vi "Polar Plat PG angle.vi"(4 "axis labels":string[](array[string])=["", "90", "180", "270"], 5 "desired font(Application)":T4(ring)=enum."Application Font", 6 "grid measurements":T1, 7 "[user-specified font]":T3, 11 "picture  in":picture) -> (3 "picture  out":picture)   [LabVIEW 2020]
panel:
  in  "label justification":T2(array[cluster])=[{"horizontal"=enum."right", "vertical"=enum."bottom"}, {"horizontal"=enum."left", "vertical"=enum."bottom"}, {"horizontal"=enum."left", "vertical"=enum."top"}, {"horizontal"=enum."right", "vertical"=enum."top"}]
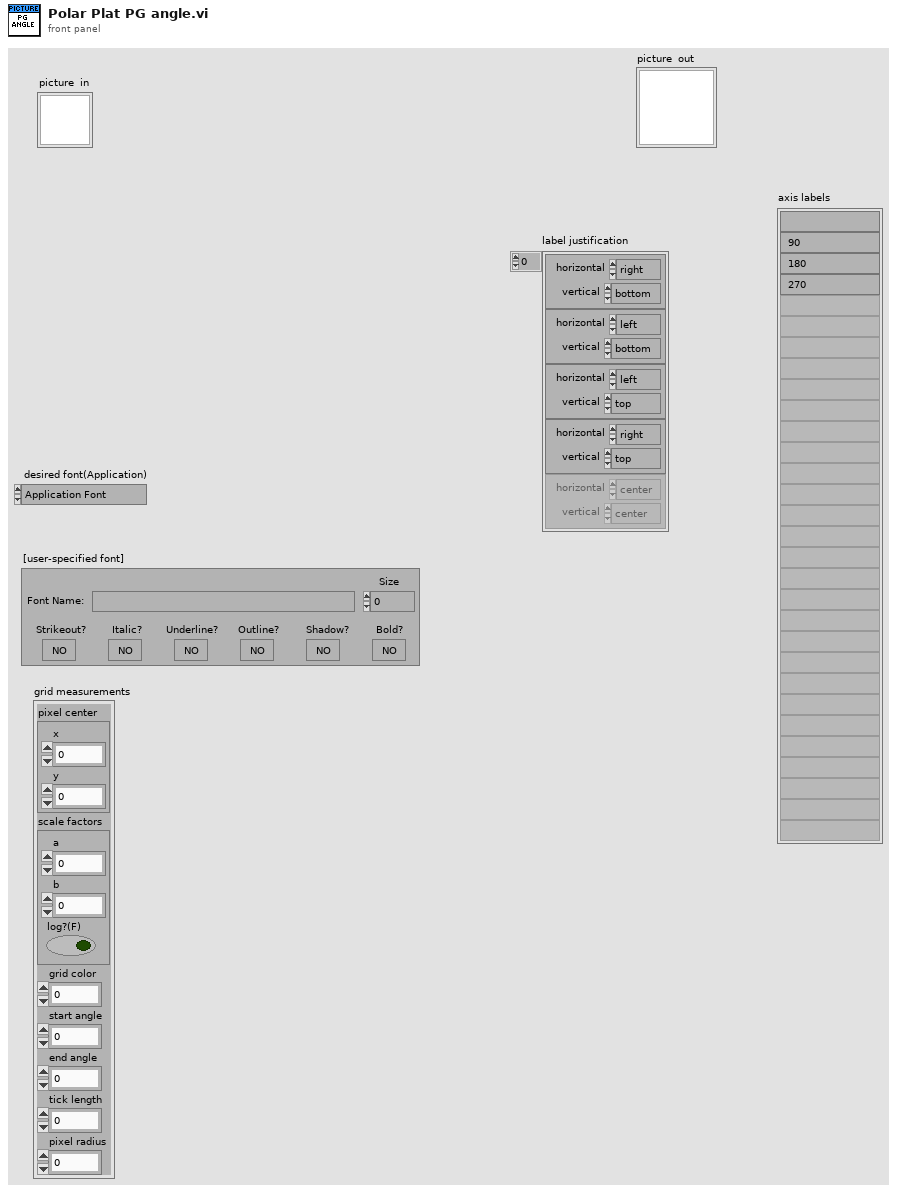
[diagram p1: front panel]
types:
  T1 = cluster{"pixel center":cluster{"x":i16, "y":i16}, "scale factors":cluster{"a":dbl, "b":dbl, "log?(F)":bool}, "grid color":u32, "start angle":dbl, "end angle":dbl, "tick length":i16, "pixel radius":i32}
  T2 = cluster{"horizontal":enum16{"left", "center", "right"}, "vertical":enum16{"top", "center", "bottom"}}[]
  T3 = cluster{"Font Name:":string, "Size":i16, "Strikeout?":bool, "Italic?":bool, "Underline?":bool, "Outline?":bool, "Shadow?":bool, "Bold?":bool}
  T4 = enum16{"User-specified Font", "Application Font", "System Font", "Dialog Font"}
  T5 = cluster{"horizontal":enum16{"left", "center", "right"}, "vertical":enum16{"top", "center", "bottom"}}
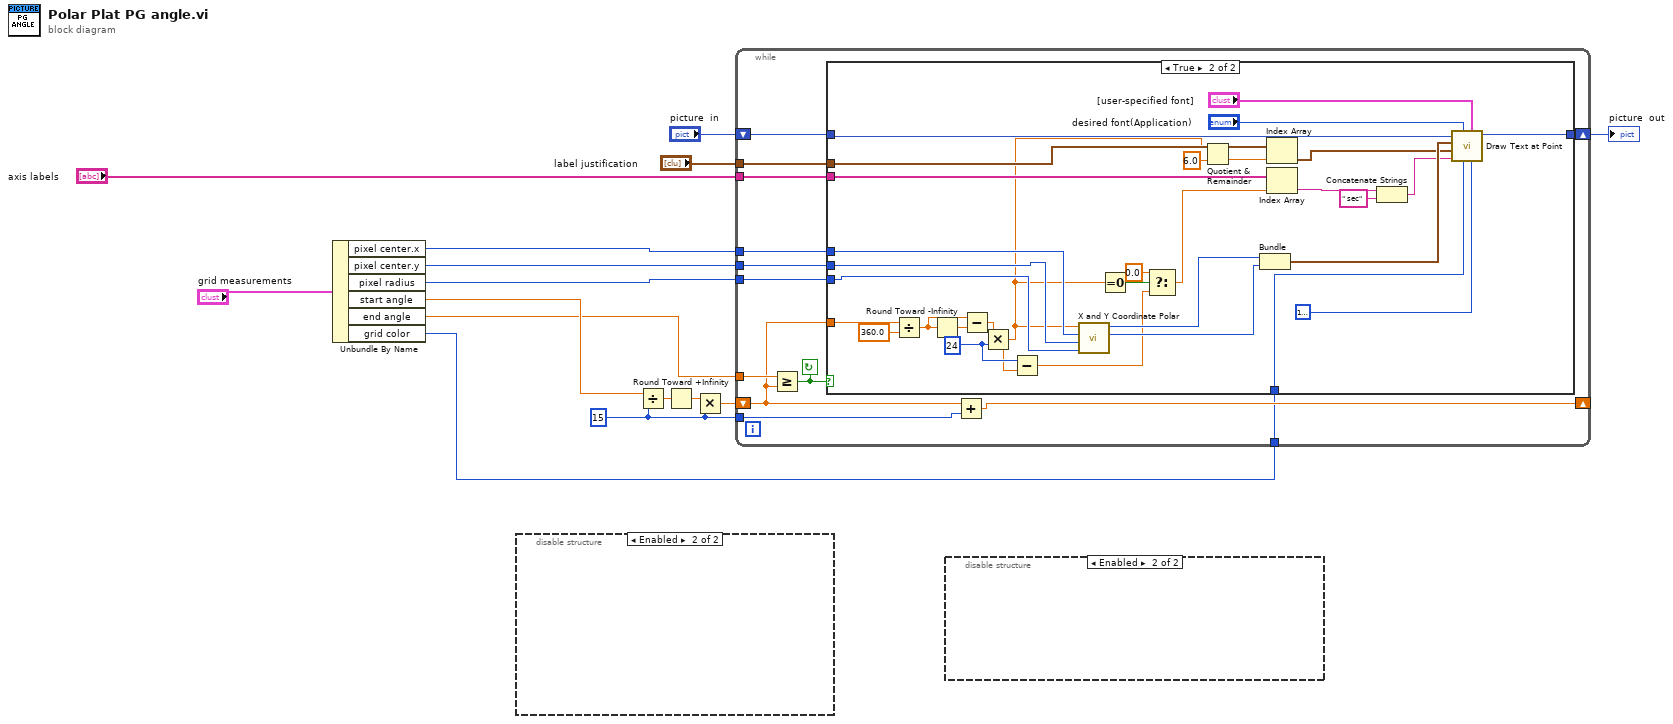
[diagram p0: block diagram]
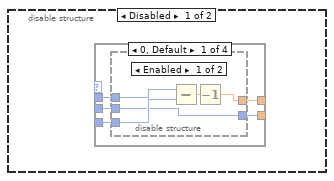
[diagram p2: hidden frame]
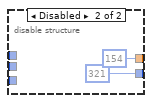
[diagram p3: hidden frame]
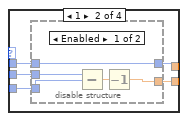
[diagram p4: hidden frame]
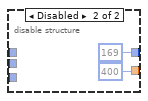
[diagram p5: hidden frame]
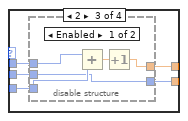
[diagram p6: hidden frame]
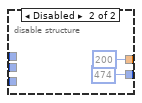
[diagram p7: hidden frame]
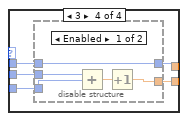
[diagram p8: hidden frame]
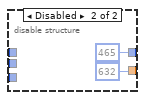
[diagram p9: hidden frame]
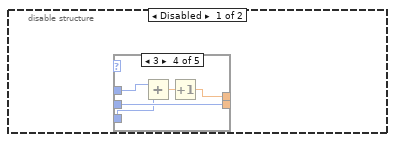
[diagram p10: hidden frame]
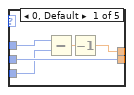
[diagram p11: hidden frame]
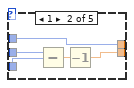
[diagram p12: hidden frame]
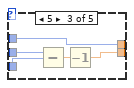
[diagram p13: hidden frame]
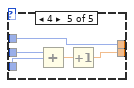
[diagram p14: hidden frame]
diagram:
  w9 = 15
  n1 = Unbundle By Name("grid measurements") -> ("pixel center.x"=w14:i16, "pixel center.y"=w13:i16, "pixel radius"=w12:i32, "start angle"=w11:dbl, "end angle"=w10:dbl, "grid color"=w15:u32)
  n2 = disable-structure shown="Enabled" {
    frame Disabled {
      n3 = case shown="0, Default" {
        selector: _ -> [_ _ _ _]
        tunnel: _ -> [w20 w29 w44 w53]
        tunnel: _ -> [w17 w32 w41 w56]
        tunnel: [w19 w28 w43 w52] -> _
        tunnel: [w16 w31 w40 w55] -> _
        tunnel: _ -> [w18 w30 w42 w54]
        frame 0, Default {
          n4 = disable-structure shown="Enabled" {
            disable-tunnel: w20 -> [w25 _]
            disable-tunnel: [w23 154] -> w19
            disable-tunnel: w18 -> [w22 _]
            disable-tunnel: w17 -> [w21 _]
            disable-tunnel: [w21 i16 321 ("y")] -> w16
            frame Enabled {
              n5 = Subtract(x=w25, y=w22) -> (x-y=w24:dbl)
              n6 = Decrement(x=w24) -> (x-1=w23:dbl)
            }
            frame Disabled {
            }
          }
        }
        frame 1 {
          n7 = disable-structure shown="Enabled" {
            disable-tunnel: w32 -> [w37 _]
            disable-tunnel: [w35 400] -> w31
            disable-tunnel: w30 -> [w34 _]
            disable-tunnel: w29 -> [w33 _]
            disable-tunnel: [w33 i16 169 ("x")] -> w28
            frame Enabled {
              n8 = Subtract(x=w37, y=w34) -> (x-y=w36:dbl)
              n9 = Decrement(x=w36) -> (x-1=w35:dbl)
            }
            frame Disabled {
            }
          }
        }
        frame 2 {
          n10 = disable-structure shown="Enabled" {
            disable-tunnel: w44 -> [w48 _]
            disable-tunnel: [w47 200] -> w43
            disable-tunnel: w42 -> [w46 _]
            disable-tunnel: w41 -> [w45 _]
            disable-tunnel: [w45 i16 474 ("y")] -> w40
            frame Enabled {
              n11 = Add(x=w48, y=w46) -> (x+y=w49:dbl)
              n12 = Increment(x=w49) -> (x+1=w47:dbl)
            }
            frame Disabled {
            }
          }
        }
        frame 3 {
          n13 = disable-structure shown="Enabled" {
            disable-tunnel: w56 -> [w61 _]
            disable-tunnel: [w59 632] -> w55
            disable-tunnel: w54 -> [w58 _]
            disable-tunnel: w53 -> [w57 _]
            disable-tunnel: [w57 i16 465 ("x")] -> w52
            frame Enabled {
              n14 = Add(x=w61, y=w58) -> (x+y=w60:dbl)
              n15 = Increment(x=w60) -> (x+1=w59:dbl)
            }
            frame Disabled {
            }
          }
        }
      }
    }
    frame Enabled {
    }
  }
  n16 = Divide(x=w11, y=w9) -> (x/y=w6:dbl)
  n17 = Round Toward +Infinity(x=w6) -> (ceil(x): smallest int >= x=w7:dbl)
  n18 = Multiply(x=w7, y=w9) -> (x*y=w8:dbl)
  n19 = while {
    tunnel: w14 -> [w67]
    tunnel: w13 -> [w68]
    tunnel: w12 -> [w69]
    shift-left: "picture  in" -> [w70]
    shift-right: [w71] -> w4
    tunnel: w10 -> [w75]
    tunnel: w9 -> [w76]
    shift-left: w8 -> [w72]
    shift-right: [w74] -> _
    tunnel: w15 -> [w66]
    tunnel: "axis labels" -> [w65]
    tunnel: "label justification" -> [w64]
    stop <- w73 continue-if-true
    n20 = Greater Or Equal?(x=w75, y=w72) -> (x >= y?=w73:bool)
    n21 = case shown="True" w73 {
      tunnel: w72 -> [_ w106]
      tunnel: [w77 w103] -> w71
      tunnel: w70 -> [w77 w102]
      tunnel: w69 -> [_ w91]
      tunnel: w68 -> [_ w92]
      tunnel: w67 -> [_ w93]
      tunnel: w66 -> [_ w99]
      tunnel: w65 -> [_ w87]
      tunnel: w64 -> [_ w86]
      frame False {
      }
      frame True {
        w88 = 24
        n22 = Divide(x=w106, y=360.0) -> (x/y=w98:dbl)
        n23 = Round Toward -Infinity(1:w98) -> (0:w108:dbl)
        n24 = Subtract(x=w98, y=w108) -> (x-y=w97:dbl)
        n25 = Multiply(x=w97, y=w88) -> (x*y=w82:dbl)
        n26 = Subtract(x=w88, y=w82) -> (x-y=w78:dbl)
        n27 = call "X and Y Coordinate Polar.vi"("Rc"=w91, "Yc"=w92, "Xc"=w93, "Selected Coordinate"=w82) -> ("Youtput"=w89:u32, "Xoutput"=w90:u32)  [unwired: 5 in, 1 out]
        n28 = Equal To 0?(x=w82) -> (x = 0?=w81:bool)
        n29 = Select(t=0.0, s=w81, f=w78) -> (s? t:f=w80:dbl)
        n30 = Quotient & Remainder(x=w82, y=6.0) -> (floor(x/y)=w84:dbl)  [unwired: 1 out]
        n31 = Bundle("Xoutput"=w90, "Youtput"=w89) -> (w104:cluster{"Xoutput":u32, "Youtput":u32})  [unwired: 1 in]
        n32 = Index Array(array=w86, index=w84) -> (element=w83:T5)
        n33 = Index Array(array=w87, index=w80) -> (element=w96:string)
        n34 = Concatenate Strings(w96, " sec" ("string")) -> (w94:string)
        n35 = call <vilib>:"Draw Text at Point.vi"("BG color(transparent)"=u32 16777216, "[user-specified font]"="[user-specified font]", "text color(black)"=w99, "desired font(Application)"="desired font(Application)", "text"=w94, "alignment(left, top)"=w83, "origin"=w104, "picture"=w102) -> ("new picture"=w103:picture)  [unwired: 2 in, 1 out]
      }
    }
    n36 = Add(x=w72, y=w76) -> (x+y=w74:dbl)
  }
  "picture  out" <- w4
  n37 = disable-structure shown="Enabled" {
    frame Disabled {
      n38 = case shown="3" {
        selector: _ -> [_ _ _ _ _]
        tunnel: _ -> [w113 w118 w123 w126 w133]
        tunnel: _ -> [w111 w117 w122 w128 w132]
        tunnel: [w110 w118 w123 w125 w133] -> _
        tunnel: [w111 w115 w120 w128 w130] -> _
        tunnel: _ -> [w109 w114 w119 w124 w129]
        frame 0, Default {
          n39 = Subtract(x=w113, y=w109) -> (x-y=w112:dbl)
          n40 = Decrement(x=w112) -> (x-1=w110:dbl)
        }
        frame 1 {
          n41 = Subtract(x=w117, y=w114) -> (x-y=w116:dbl)
          n42 = Decrement(x=w116) -> (x-1=w115:dbl)
        }
        frame 5 {
          n43 = Subtract(x=w122, y=w119) -> (x-y=w121:dbl)
          n44 = Decrement(x=w121) -> (x-1=w120:dbl)
        }
        frame 3 {
          n45 = Add(x=w126, y=w124) -> (x+y=w127:dbl)
          n46 = Increment(x=w127) -> (x+1=w125:dbl)
        }
        frame 4 {
          n47 = Add(x=w132, y=w129) -> (x+y=w131:dbl)
          n48 = Increment(x=w131) -> (x+1=w130:dbl)
        }
      }
    }
    frame Enabled {
    }
  }
